vi "closeCanon.vi"(8 "error in":errorcluster, 11 "inCameraRef":u32=4294967295) -> ()   [LabVIEW 2016]
panel:
  out "error out":errorcluster
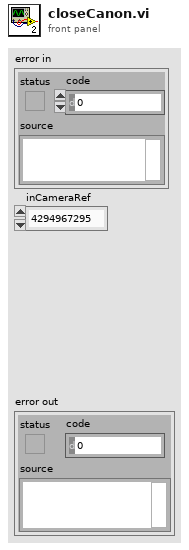
[diagram p1: front panel]
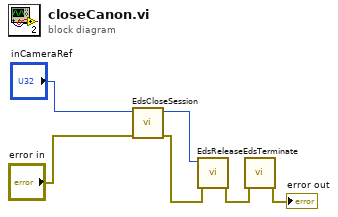
[diagram p0: block diagram]
diagram:
  n1 = call "EdsCloseSession.vi"("error in"="error in", "inCameraRef"="inCameraRef") -> ("error out"=w6:errorcluster, "inCameraRef dup"=w3:u32)  [unwired: 8 in]
  n2 = call "EdsRelease.vi"("error in"=w6, "inRef"=w3) -> ("error out"=w4:errorcluster)  [unwired: 7 in, 2 out]
  n3 = call "EdsTerminate.vi"("error in"=w4) -> ("error out"=→"error out":errorcluster)  [unwired: 10 in]
